vi "Global var FPGA.vi"() -> ()   [LabVIEW 2020]
panel:
  out "Updated Weights and Biases":sgl[](array[numeric])
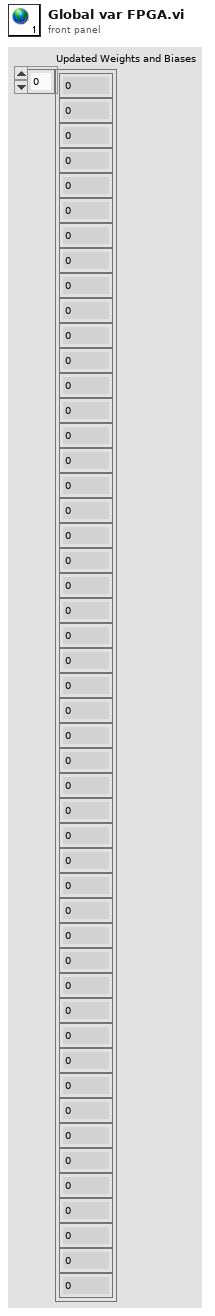
[diagram p1: front panel]
diagram:
